vi "Initialize.vi"(8 "error in (no error)":errorcluster, 11 "View Template in":refnum<class "Normal Log.lvclass">) -> (0 "error out":errorcluster, 3 "View Template out":refnum<class "Normal Log.lvclass">)   [LabVIEW 2020, in "Normal Log.lvlib" / "Normal Log.lvclass"]
uses:
  Normal Log.lvclass
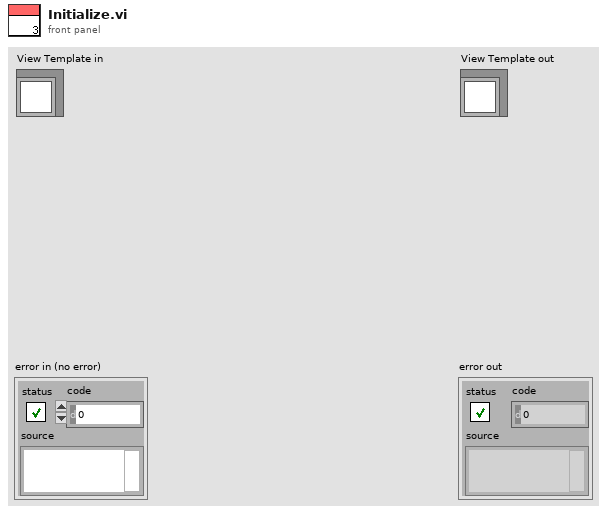
[diagram p1: front panel]
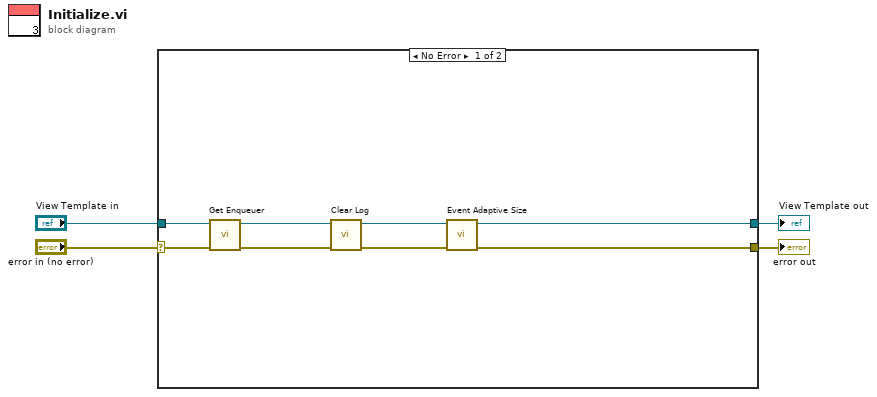
[diagram p0: block diagram]
diagram:
  n1 = case shown="No Error" "error in (no error)" {
    selector: "error in (no error)" -> [w11 w14]
    tunnel: [w10 w14] -> w3
    tunnel: [w9 w13] -> w1
    tunnel: "View Template in" -> [w12 w13]
    frame No Error {
      n2 = call "Get Enqueuer.vi"("error in (no error)"=w11, "View Template in"=w12) -> ("error out"=w6:errorcluster, "View Template out"=w8:refnum<class "Normal Log.lvclass">)  [unwired: 8 in]
      n3 = call "Clear Log.vi"("error in (no error)"=w6, "Normal Log in"=w8) -> ("error out"=w5:errorcluster, "Normal Log out"=w7:refnum<class "Normal Log.lvclass">)  [unwired: 8 in]
      n4 = call "Event Adaptive Size.vi"("error in (no error)"=w5, "Normal Log in"=w7) -> ("error out"=w10:errorcluster, "Normal Log out"=w9:refnum<class "Normal Log.lvclass">)  [unwired: 8 in]
    }
    frame Error {
    }
  }
  "error out" <- w3
  "View Template out" <- w1
